vi "BuildMacro.vi"(0 "instrument handle":refnum<visa-resource-name>, 1 "Hold time (s)":sgl, 2 "Current Test":i32, 3 "# Tests":i32, 4 "Periods/test":i32, 5 "error in":errorcluster, 6 "Test type":string(combo)="Voltage", 7 "Enable NHR?":bool) -> (12 "Macro file string":string, 14 "instrument handle out":refnum<visa-resource-name>, 15 "Max Current":dbl, 16 "Max Voltage":dbl, 17 "Test time":dbl, 19 "error out":errorcluster)   [LabVIEW 2018]
uses:
  <vilib>/Utility/error.llb/DialogType.ctl
  <instrlib>/NHRDCPowerModule/NHRDCPowerModule/NHRDCPowerModule.lvlib
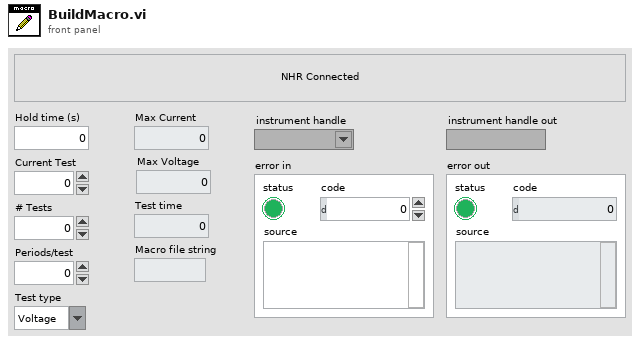
[diagram p1: front panel]
types:
  T1 = typedef "DialogType.ctl" = u16
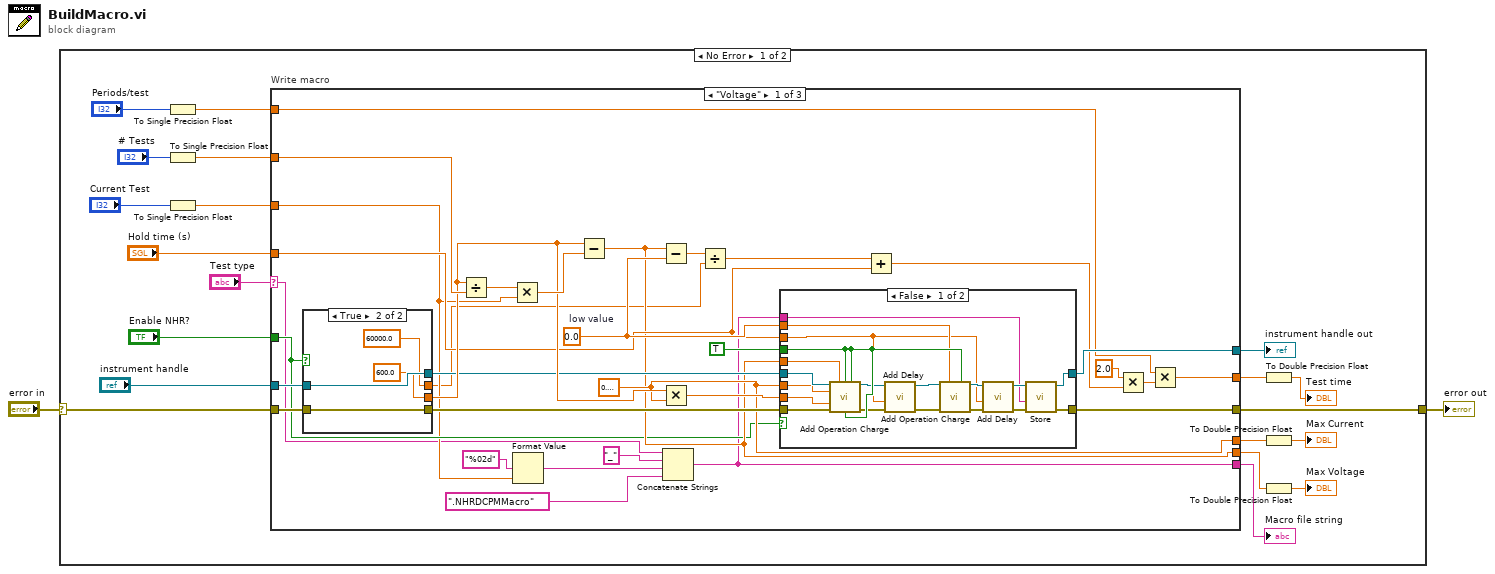
[diagram p0: block diagram]
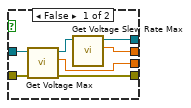
[diagram p3: hidden frame]
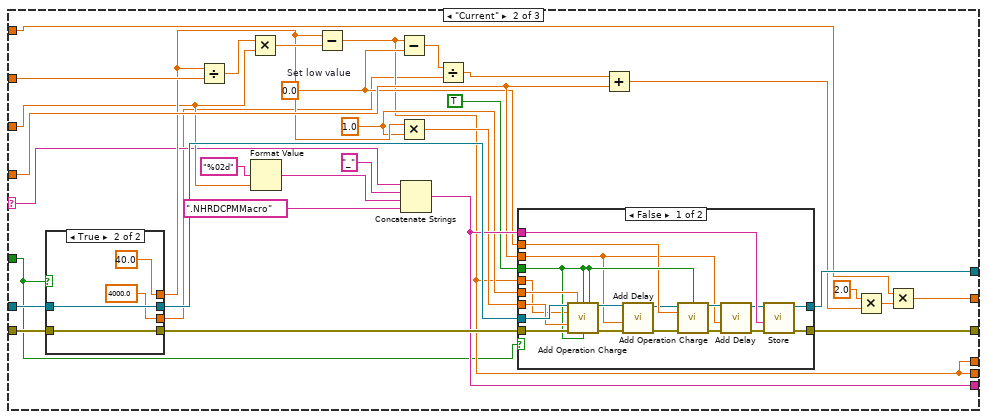
[diagram p4: hidden frame]
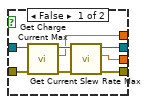
[diagram p6: hidden frame]
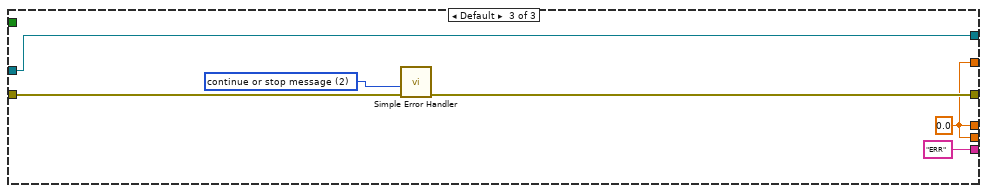
[diagram p7: hidden frame]
diagram:
  n1 = case shown="No Error" "error in" {
    selector: "error in" -> [w10 w158]
    tunnel: [w19 w158] -> w2
    frame No Error {
      n2 = To Single Precision Float(number="Periods/test") -> (single precision float=w9:sgl)
      n3 = To Single Precision Float(number="# Tests") -> (single precision float=w8:sgl)
      n4 = To Single Precision Float(number="Current Test") -> (single precision float=w7:sgl)
      n5 = case "Write macro" shown="\"Voltage\"" "Test type" {
        selector: "Test type" -> [w23 w88 _]
        tunnel: "Hold time (s)" -> [w41 w106 _]
        tunnel: w8 -> [w54 w118 _]
        tunnel: w7 -> [w25 w91 _]
        tunnel: "instrument handle" -> [w32 w114 w152]
        tunnel: [w46 w111 w152] -> w21
        tunnel: [w45 w110 w155] -> w19
        tunnel: [w26 w109 "ERR"] -> w20
        tunnel: w9 -> [w37 w102 _]
        tunnel: [w36 w100 w154] -> w22
        tunnel: [w35 w94 w154] -> w18
        tunnel: [w34 w94 w154] -> w12
        tunnel: w10 -> [w33 w101 w157]
        tunnel: "Enable NHR?" -> [w31 w93 _]
        frame "Voltage" {
          w44 = sgl 0.0  # low value
          w35 = sgl 0.1 ("current (0.0)")
          n6 = case shown="True" w31 {
            tunnel: [w82 sgl 600.0 ("maximum voltage")] -> w52
            tunnel: [w77 w85] -> w50
            tunnel: [w80 w86] -> w49
            tunnel: w33 -> [w79 w86]
            tunnel: w32 -> [w78 w85]
            tunnel: [w76 sgl 60000.0 ("maximum voltage slew rate")] -> w24
            frame False {
              n7 = call <instrlib>:"Get Voltage Max.vi"("error in (no error)"=w79, "instrument handle"=w78) -> ("error out"=w80:errorcluster, "maximum voltage"=w82:sgl, "instrument handle out"=w81:refnum<visa-resource-name>)  [unwired: 7 in]
              n8 = call <instrlib>:"Get Voltage Slew Rate Max.vi"("instrument handle"=w81) -> ("maximum voltage slew rate"=w76:sgl, "instrument handle out"=w77:refnum<visa-resource-name>)  [unwired: 8 in, 1 out]
            }
            frame True {
            }
          }
          n9 = Divide ("calculate inter-test step")(x=w52, y=w54) -> (x/y=w47:sgl)
          n10 = Multiply(x=w47, y=w25) -> (x*y=w53:sgl)
          n11 = Format Value(format string="%02d", value (0)=w25) -> (output string=w27:string)  [unwired: 1 in]
          n12 = Subtract ("calculate high value")(x=w52, y=w53) -> (x-y=w34:sgl)
          n13 = Subtract ("calculate delta")(x=w34, y=w44) -> (x-y=w43:sgl)
          n14 = Multiply ("Get Power")(x=w52, y=w35) -> (x*y=w51:sgl)
          n15 = Concatenate Strings(w23, "_" ("string"), w27, ".NHRDCPMMacro" ("string")) -> (w26:string)
          n16 = Divide ("slew time (s)")(x=w43, y=w24) -> (x/y=w42:sgl)
          n17 = case shown="False" w31 {
            tunnel: w51 -> [w73 _]
            tunnel: w50 -> [w72 w75]
            tunnel: w49 -> [w71 w74]
            tunnel: TRUE ("use current (false)") -> [w70 _]
            tunnel: [w69 w75] -> w46
            tunnel: [w68 w74] -> w45
            tunnel: w44 -> [w67 _]
            tunnel: w41 -> [w55 _]
            tunnel: w35 -> [w66 _]
            tunnel: w34 -> [w65 _]
            tunnel: w26 -> [w56 _]
            frame False {
              n18 = call <instrlib>:"Add Operation Charge.vi"("instrument handle"=w72, "voltage (0.0)"=w65, "use current (false)"=w70, "use voltage (false)"=w70, "current (0.0)"=w66, "power (0.0)"=w73, "error in (no error)"=w71, "use power (false)"=w70) -> ("instrument handle out"=w64:refnum<visa-resource-name>, "error out"=w63:errorcluster)  [unwired: 6 in]
              n19 = call <instrlib>:"Add Delay.vi"("error in (no error)"=w63, "delay (0.0)"=w55, "instrument handle"=w64) -> ("error out"=w61:errorcluster, "instrument handle out"=w62:refnum<visa-resource-name>)  [unwired: 7 in]
              n20 = call <instrlib>:"Add Operation Charge.vi"("instrument handle"=w62, "voltage (0.0)"=w67, "use voltage (false)"=w70, "error in (no error)"=w61) -> ("instrument handle out"=w59:refnum<visa-resource-name>, "error out"=w60:errorcluster)  [unwired: 10 in]
              n21 = call <instrlib>:"Add Delay.vi"("error in (no error)"=w60, "delay (0.0)"=w55, "instrument handle"=w59) -> ("error out"=w57:errorcluster, "instrument handle out"=w58:refnum<visa-resource-name>)  [unwired: 7 in]
              n22 = call <instrlib>:"Store.vi"("error in (no error)"=w57, "path (\"\")"=w56, "instrument handle"=w58) -> ("error out"=w68:errorcluster, "instrument handle out"=w69:refnum<visa-resource-name>)  [unwired: 7 in]
            }
            frame True {
            }
          }
          n23 = Add(x=w42, y=w41) -> (x+y=w40:sgl)
          n24 = Multiply ("single wave period")(x=sgl 2.0, y=w40) -> (x*y=w38:sgl)
          n25 = Multiply ("test period")(x=w37, y=w38) -> (x*y=w36:sgl)
        }
        frame "Current" {
          w97 = sgl 1.0 ("voltage (0.0)")
          w95 = sgl 0.0  # Set low value
          n26 = case shown="True" w93 {
            tunnel: [w143 w150] -> w116
            tunnel: [w141 w151] -> w115
            tunnel: w114 -> [w146 w150]
            tunnel: w101 -> [w145 w151]
            tunnel: [w144 sgl 40.0 ("charge current max")] -> w99
            tunnel: [w140 sgl 4000.0 ("maximum current slew rate")] -> w87
            frame False {
              n27 = call <instrlib>:"Get Charge Current Max.vi"("error in (no error)"=w145, "instrument handle"=w146) -> ("error out"=w142:errorcluster, "charge current max"=w144:sgl, "instrument handle out"=w147:refnum<visa-resource-name>)  [unwired: 7 in]
              n28 = call <instrlib>:"Get Current Slew Rate Max.vi"("error in (no error)"=w142, "instrument handle"=w147) -> ("error out"=w141:errorcluster, "maximum current slew rate"=w140:sgl, "instrument handle out"=w143:refnum<visa-resource-name>)  [unwired: 7 in]
            }
            frame True {
            }
          }
          n29 = Divide ("calculate inter-test step")(x=w99, y=w118) -> (x/y=w113:sgl)
          n30 = Multiply(x=w113, y=w91) -> (x*y=w117:sgl)
          n31 = Format Value(format string="%02d", value (0)=w91) -> (output string=w89:string)  [unwired: 1 in]
          n32 = Subtract ("calculate high value")(x=w99, y=w117) -> (x-y=w94:sgl)
          n33 = Subtract ("calculate delta")(x=w94, y=w95) -> (x-y=w108:sgl)
          n34 = Multiply ("Get Power")(x=w99, y=w97) -> (x*y=w98:sgl)
          n35 = Concatenate Strings(w88, "_" ("string"), w89, ".NHRDCPMMacro" ("string")) -> (w109:string)
          n36 = Divide ("slew time (s)")(x=w108, y=w87) -> (x/y=w107:sgl)
          n37 = case shown="False" w93 {
            tunnel: w116 -> [w137 w138]
            tunnel: w115 -> [w136 w139]
            tunnel: [w135 w138] -> w111
            tunnel: [w134 w139] -> w110
            tunnel: w109 -> [w133 _]
            tunnel: w106 -> [w119 _]
            tunnel: w98 -> [w132 _]
            tunnel: w97 -> [w131 _]
            tunnel: TRUE ("use current (false)") -> [w130 _]
            tunnel: w95 -> [w129 _]
            tunnel: w94 -> [w128 _]
            frame False {
              n38 = call <instrlib>:"Add Operation Charge.vi"("instrument handle"=w137, "voltage (0.0)"=w131, "use current (false)"=w130, "use voltage (false)"=w130, "current (0.0)"=w128, "power (0.0)"=w132, "error in (no error)"=w136, "use power (false)"=w130) -> ("instrument handle out"=w127:refnum<visa-resource-name>, "error out"=w126:errorcluster)  [unwired: 6 in]
              n39 = call <instrlib>:"Add Delay.vi"("error in (no error)"=w126, "delay (0.0)"=w119, "instrument handle"=w127) -> ("error out"=w124:errorcluster, "instrument handle out"=w125:refnum<visa-resource-name>)  [unwired: 7 in]
              n40 = call <instrlib>:"Add Operation Charge.vi"("instrument handle"=w125, "use current (false)"=w130, "current (0.0)"=w129, "error in (no error)"=w124) -> ("instrument handle out"=w122:refnum<visa-resource-name>, "error out"=w123:errorcluster)  [unwired: 10 in]
              n41 = call <instrlib>:"Add Delay.vi"("error in (no error)"=w123, "delay (0.0)"=w119, "instrument handle"=w122) -> ("error out"=w120:errorcluster, "instrument handle out"=w121:refnum<visa-resource-name>)  [unwired: 7 in]
              n42 = call <instrlib>:"Store.vi"("error in (no error)"=w120, "path (\"\")"=w133, "instrument handle"=w121) -> ("error out"=w134:errorcluster, "instrument handle out"=w135:refnum<visa-resource-name>)  [unwired: 7 in]
            }
            frame True {
            }
          }
          n43 = Add(x=w107, y=w106) -> (x+y=w105:sgl)
          n44 = Multiply ("single wave period")(x=sgl 2.0, y=w105) -> (x*y=w103:sgl)
          n45 = Multiply ("test period")(x=w102, y=w103) -> (x*y=w100:sgl)
        }
        frame Default {
          w154 = sgl 0.0
          w156 = T1 2 items=["no dialog", "OK message", "continue or stop message", "OK message + warnings", "continue/stop + warnings"] ("type of dialog (OK msg:1)")
          n46 = call <vilib>:"Simple Error Handler.vi"("type of dialog (OK msg:1)"=w156, "error in (no error)"=w157) -> ("error out"=w155:errorcluster)  [unwired: 3 in, 4 out]
        }
      }
      "instrument handle out" <- w21
      "Macro file string" <- w20
      n47 = To Double Precision Float(number=w22) -> (double precision float=→"Test time":dbl)
      n48 = To Double Precision Float(number=w18) -> (double precision float=→"Max Current":dbl)
      n49 = To Double Precision Float(number=w12) -> (double precision float=→"Max Voltage":dbl)
    }
    frame Error {
    }
  }
  "error out" <- w2
